vi "UpdatePalette.vi"(0 "palette path":path, 2 "SubmenuPath":path, 5 "error in (no error)":errorcluster) -> (19 "error out":errorcluster)   [LabVIEW 2020, in "G#Installer.lvlib"]
uses:
  G#Installer.lvlib
  <vilib>/Palette API/Palette Menu/Public Type Define/Palette type.ctl
  <vilib>/Palette API/Palette Menu/Public Type Define/Item.ctl
  <vilib>/Palette API/Palette Menu/Palette Menu.lvlib
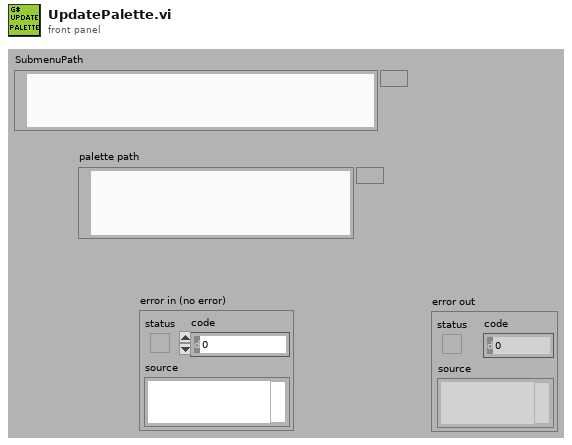
[diagram p1: front panel]
types:
  T1 = typedef "Palette Menu.lvlib/Item.ctl" = cluster{"item path":path, "library path":path, "use default lvlib palette":bool, "short name":string, "place VI contents":bool, "hide synchronized item":bool, "reserve spot for synch item":bool, "configure when placing VI contents":bool}
  T2 = typedef "Palette Menu.lvlib/Palette type.ctl" = i32
  T3 = typedef "Palette Menu.lvlib/Palette Data.ctl" = cluster{"display name":string, "view format":T4, "palette width":i16, "items":T5, "256 color icon":picture, "B&W color icon":picture, "help information":T6, "palette description":string, "synchronize information":T7}
  T4 = typedef "Palette Menu.lvlib/View Format.ctl" = u16
  T5 = typedef "Palette Menu.lvlib/Items.ctl" = T1[]
  T6 = typedef "Palette Menu.lvlib/Help Info.ctl" = cluster{"help tag":string, "help file path ":path}
  T7 = typedef "Palette Menu.lvlib/Synchronize Info.ctl" = cluster{"synchronize with directory":bool, "synchronize directory path":path}
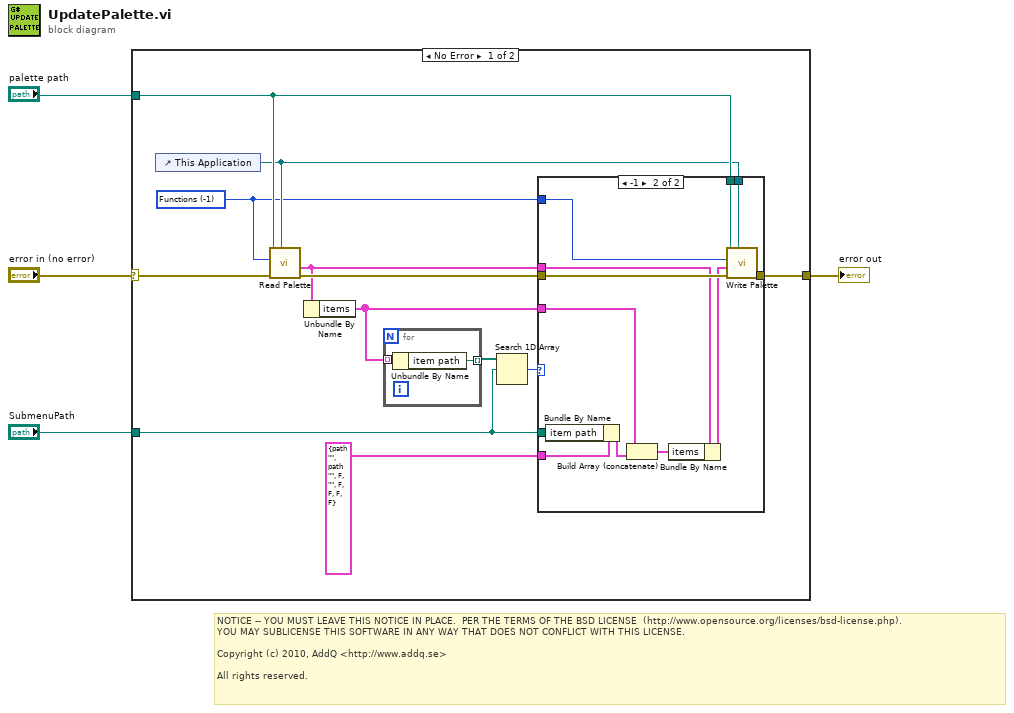
[diagram p0: block diagram]
diagram:
  # "NOTICE -- YOU MUST LEAVE THIS NOTICE IN PLACE.  PER THE TERMS OF THE BSD LICENSE  (http://www.opensource.org/licenses/bsd-license.php).\nYOU MAY SUBLICENSE THIS SOFTWARE IN ANY WAY THAT DOES NOT CONFLICT WITH THIS LICENSE.\n\nCopyright (c) 2010, AddQ <http://www.addq.se>\n\nAll rights reserved."
  n1 = case shown="No Error" "error in (no error)" {
    selector: "error in (no error)" -> [w9 w32]
    tunnel: "SubmenuPath" -> [w6 _]
    tunnel: "palette path" -> [w16 _]
    tunnel: [w10 w32] -> w2
    frame No Error {
      w13 = T2 -1 items=["Functions"=-1, "Controls"=-2] ("palette type")
      n2 = control-ref of="This Application"() -> (w15:refnum<vi>)
      n3 = call <vilib>:"Read Palette.vi"("application reference"=w15, "error in (no error)"=w9, "palette type"=w13, "palette path"=w16) -> ("error out"=w14:errorcluster, "palette data"=w12:T3)  [unwired: 5 in, 1 out]
      n4 = Unbundle By Name(w12) -> ("items"=w8:T5)
      n5 = for {
        tunnel: w8 -> [w31] mode=indexing
        tunnel: [w30] -> w7 mode=indexing
        n6 = Unbundle By Name(w31) -> ("item path"=w30:path)
      }
      n7 = Search 1D Array(1D array=w7, element=w6) -> (index of element=w5:i32)  [unwired: 1 in]
      n8 = case shown="-1" w5 {
        tunnel: w16 -> [_ w29]
        tunnel: w15 -> [_ w28]
        tunnel: w14 -> [w17 w27]
        tunnel: w13 -> [_ w26]
        tunnel: w12 -> [_ w25]
        tunnel: T1 {"item path"=path "", "library path"=path "", "use default lvlib palette"=FALSE, "short name"="", "place VI contents"=FALSE, "hide synchronized item"=FALSE, "reserve spot for synch item"=FALSE, "configure when placing VI contents"=FALSE} ("Items") -> [_ w22]
        tunnel: [w17 w20] -> w10
        tunnel: w8 -> [_ w19]
        tunnel: w6 -> [_ w18]
        frame Default {
          # "Already installed"
        }
        frame -1 {
          n9 = Bundle By Name(cluster=w22, "item path"=w18) -> (w21:T1)
          n10 = Build Array (concatenate)(w19, w21) -> (w23:T5)
          n11 = Bundle By Name(cluster=w25, "items"=w23) -> (w24:T3)
          n12 = call <vilib>:"Write Palette.vi"("application reference"=w28, "error in (no error)"=w27, "palette data"=w24, "palette type"=w26, "palette path"=w29) -> ("error out"=w20:errorcluster)  [unwired: 6 in]
        }
      }
    }
    frame Error {
    }
  }
  "error out" <- w2
